vi "Set Type.vi"(10 "Type":refnum<class "Type.lvclass">, 11 "DoublePanel in":refnum<class "DoublePanel.lvclass">) -> (3 "DoublePanel out":refnum<class "DoublePanel.lvclass">)   [LabVIEW 2020, in "Conditum-Tools.lvlib" / "DoublePanel.lvclass"]
uses:
  DoublePanel.lvclass
  Conditum-Clone/Columns/Type/Type.lvclass
  DoublePanel.lvclass/DoublePanel.ctl
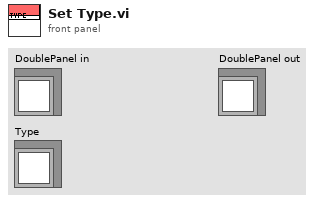
[diagram p1: front panel]
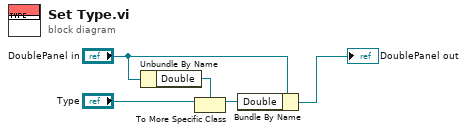
[diagram p0: block diagram]
diagram:
  n1 = Unbundle By Name("DoublePanel in") -> ("Double"=w3:refnum<class "Double.lvclass">)
  n2 = To More Specific Class(target class=w3, reference="Type") -> (specific class reference=w2:refnum<class "Double.lvclass">)  [unwired: 1 in, 1 out]
  n3 = Bundle By Name(cluster="DoublePanel in", "Double"=w2) -> (→"DoublePanel out":refnum<class "DoublePanel.lvclass">)
